vi "P3_Com_Datos_SCOF.vi"() -> ()   [LabVIEW 2019]
uses:
  <vilib>/Instr/_visa.llb/VISA Set IO Buffer Mask.ctl
  <vilib>/Analysis/baseanly.llb/Mean (DBL).vi
  <vilib>/Instr/_visa.llb/VISA Configure Serial Port (Instr).vi
  <vilib>/Analysis/NI_AALBase.lvlib
panel:
  out "Promedio RPM":dbl format="%0.2f"
  out "Grafica de Velocidad":dbl[][](graph)
  in  "Set Point":dbl(slide) scale=0.0..3000.0
  out "rpm":dbl
  out "strv":i32
  out "return count":u32
  out "read buffer":string
  in  "baud rate (9600)":u32=115200
  in  "VISA resource name":refnum<visa-resource-name>="COM3"
  in  "stop":bool
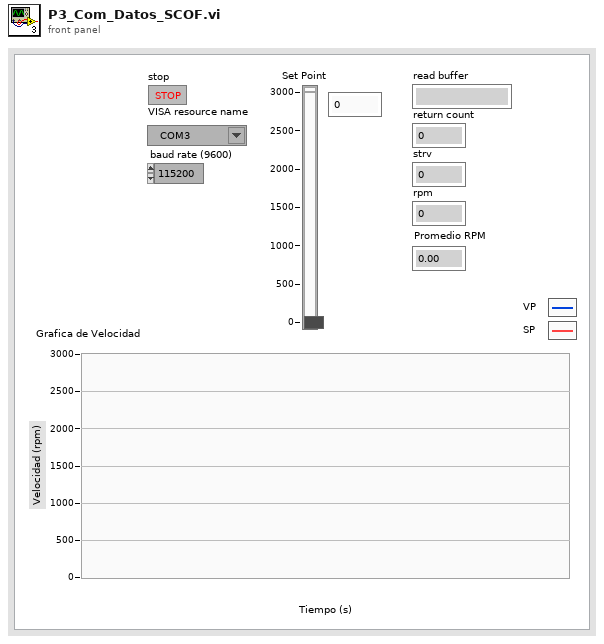
[diagram p1: front panel]
types:
  T1 = typedef "VISA Set IO Buffer Mask.ctl" = u16
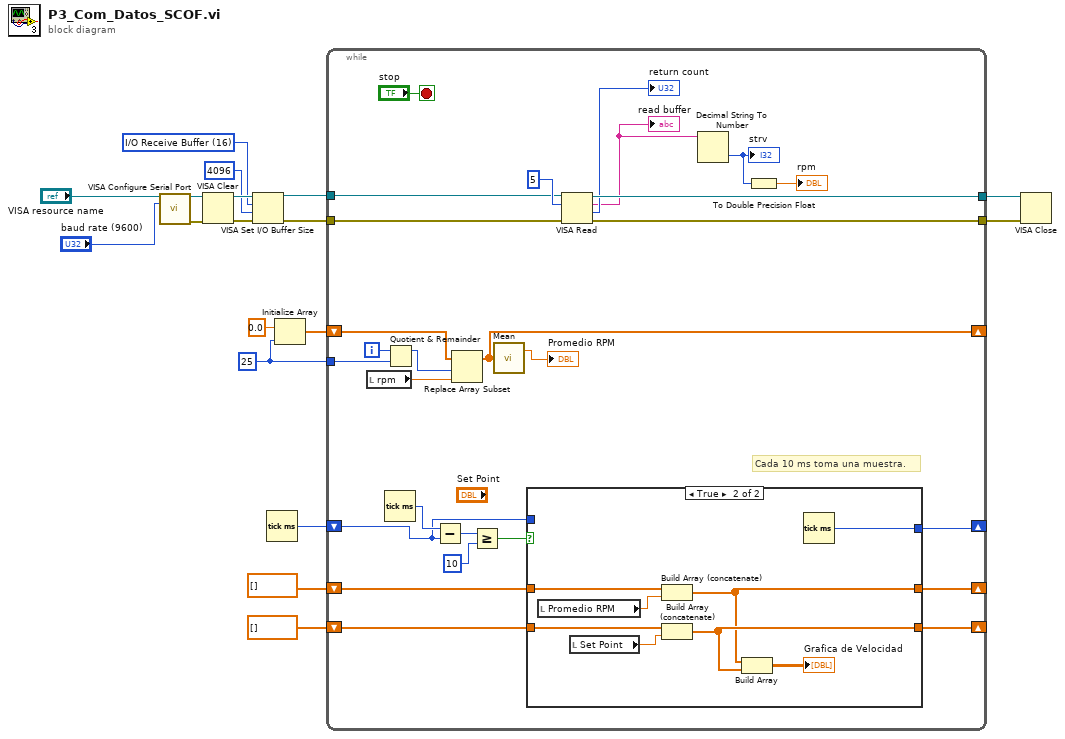
[diagram p0: block diagram]
diagram:
  w1 = 25 ("Tamaño Vppi")
  w10 = T1 16 items=["I/O Receive Buffer"=16, "I/O Transmit Buffer"=32, "I/O Receive and Transmit Buffer"=48] ("Mask")
  n1 = call-poly "VISA Configure Serial Port"("VISA resource name"="VISA resource name", "baud rate (9600)"="baud rate (9600)") -> ("VISA resource name out"=w14:refnum<visa-resource-name>, "error out"=w13:errorcluster)  [unwired: 12 in]
  n2 = VISA Clear(VISA resource name=w14, error in (no error)=w13) -> (VISA resource name out=w12:refnum<visa-resource-name>, error out=w11:errorcluster)
  n3 = VISA Set I/O Buffer Size(VISA resource name=w12, mask (16)=w10, size (4096)=u32 4096, error in (no error)=w11) -> (VISA resource name out=w8:refnum<visa-resource-name>, error out=w7:errorcluster)
  n4 = Tick Count (ms)() -> (millisecond timer value=w6:u32)
  n5 = Initialize Array(0.0 ("element"), w1) -> (w2:dbl[])
  n6 = while {
    tunnel: [w44] -> w18
    tunnel: [w43] -> w17
    tunnel: w8 -> [w41]
    tunnel: w7 -> [w40]
    shift-right: [w29] -> _
    shift-left: w6 -> [w32]
    shift-right: [w28] -> _
    shift-left: dbl[] [] -> [w31]
    shift-right: [w27] -> _
    shift-left: dbl[] [] -> [w30]
    tunnel: w1 -> [w23]
    shift-right: [w21] -> _
    shift-left: w2 -> [w25]
    i -> [w24]
    stop <- "stop" stop-if-true
    # "Cada 10 ms toma una muestra."
    n7 = local read "rpm"() -> (w22:dbl)
    n8 = Tick Count (ms)() -> (millisecond timer value=w33:u32)
    n9 = Quotient & Remainder(x=w24, y=w23) -> (x-y*floor(x/y)=w26:i32)  [unwired: 1 out]
    n10 = Subtract(x=w33, y=w32) -> (x-y=w34:u32)
    n11 = Replace Array Subset(array=w25, new element=w22, index=w26) -> (w21:dbl[])
    n12 = Greater Or Equal?(x=w34, y=u32 10) -> (x >= y?=w35:bool)
    n13 = call-poly <vilib>:"Mean.vi"("X"=w21) -> ("mean"=→"Promedio RPM":dbl)  [unwired: 1 out]
    n14 = case shown="True" w35 {
      tunnel: [w48 w56] -> w29
      tunnel: w32 -> [w48 _]
      tunnel: w31 -> [w47 w55]
      tunnel: w30 -> [w46 w54]
      tunnel: [w47 w49] -> w28
      tunnel: [w46 w51] -> w27
      frame False {
      }
      frame True {
        n15 = local read "Promedio RPM"() -> (w53:dbl)
        n16 = local read "Set Point"() -> (w52:dbl)
        n17 = Build Array (concatenate)(w55, w53) -> (w49:dbl[])
        n18 = Build Array (concatenate)(w54, w52) -> (w51:dbl[])
        n19 = Build Array(w49, w51) -> (→"Grafica de Velocidad":dbl[][])
        n20 = Tick Count (ms)() -> (millisecond timer value=w56:u32)
      }
    }
    n21 = VISA Read(VISA resource name=w41, byte count=u32 5, error in (no error)=w40) -> (VISA resource name out=w44:refnum<visa-resource-name>, read buffer=w38:string, return count=→"return count":u32, error out=w43:errorcluster)
    "read buffer" <- w38
    n22 = Decimal String To Number(string=w38) -> (number=w37:i32)  [unwired: 2 in, 1 out]
    "strv" <- w37
    n23 = To Double Precision Float(number=w37) -> (double precision float=→"rpm":dbl)
  }
  n24 = VISA Close(VISA resource name=w18, error in (no error)=w17) -> ()  [unwired: 1 out]
